vi "panel_update_status_string.vi"(8 "error in (no error)":errorcluster, 10 "String":string, 11 "newport_xps_panel in":refnum<class "newport_xps_panel.lvclass">) -> (0 "error out":errorcluster, 3 "newport_xps_panel out":refnum<class "newport_xps_panel.lvclass">)   [LabVIEW 2015, in "newport_xps_panel.lvclass"]
uses:
  newport_xps_panel.lvclass
  newport_xps_panel.lvclass/newport_xps_panel.ctl
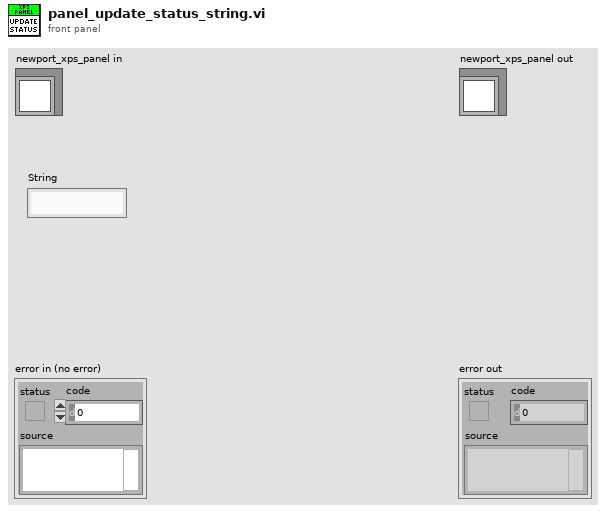
[diagram p1: front panel]
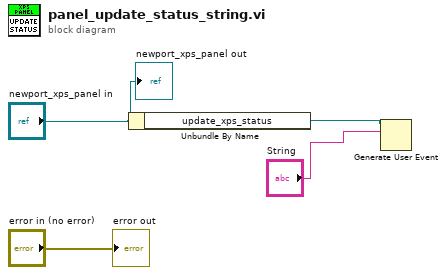
[diagram p0: block diagram]
diagram:
  n1 = Unbundle By Name("newport_xps_panel in") -> ("update_xps_status"=w2:refnum<user-event>)
  n2 = Generate User Event(user event=w2, event data cluster="String") -> ()  [unwired: 2 in, 2 out]
  "error out" <- "error in (no error)"
  "newport_xps_panel out" <- "newport_xps_panel in"
